vi "DateTimeString.vi"() -> (3 "date/time string":string)   [LabVIEW 2014]
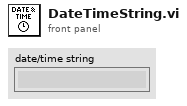
[diagram p1: front panel]
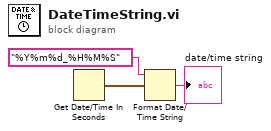
[diagram p0: block diagram]
diagram:
  n1 = Get Date/Time In Seconds() -> (seconds since 1Jan1904=w3:timestamp)
  n2 = Format Date/Time String(time format string (%c)="%Y%m%d_%H%M%S", seconds (now)=w3) -> (date/time string=→"date/time string":string)  [unwired: 1 in]
